vi "应到角度.vi"(1 "目前位置":cluster{"x（cm）":dbl, "y（cm）":dbl, "角度（度）":dbl}, 2 "目标位置":cluster{"x（cm）":dbl, "y（cm）":dbl, "角度（度）":dbl}) -> (0 "应到角度":dbl format="%#_13g")   [LabVIEW 2016]
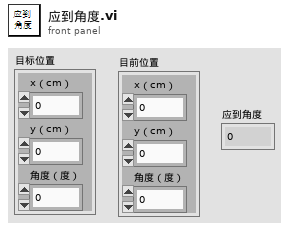
[diagram p1: front panel]
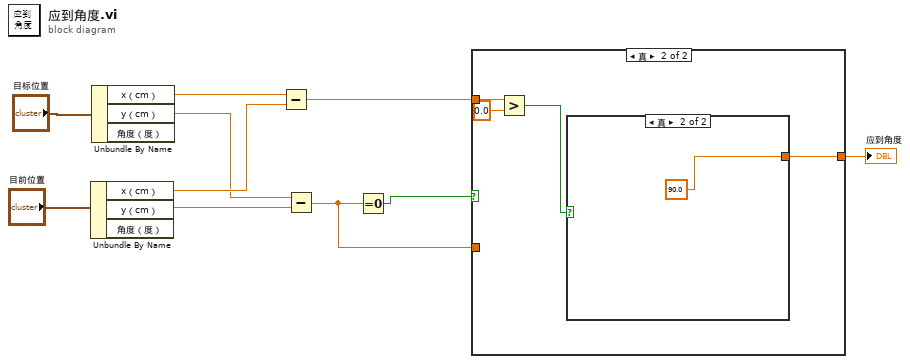
[diagram p0: block diagram]
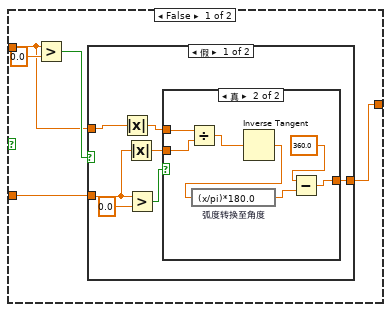
[diagram p2: hidden frame]
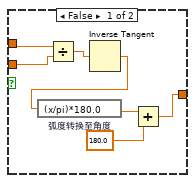
[diagram p3: hidden frame]
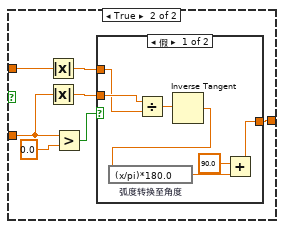
[diagram p4: hidden frame]
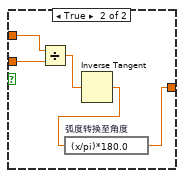
[diagram p5: hidden frame]
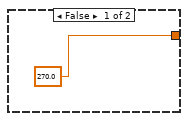
[diagram p6: hidden frame]
diagram:
  n1 = Unbundle By Name("目前位置") -> ("x（cm）"=w7:dbl, "y（cm）"=w5:dbl)  [unwired: 1 out]
  n2 = Unbundle By Name("目标位置") -> ("x（cm）"=w8:dbl, "y（cm）"=w6:dbl)  [unwired: 1 out]
  n3 = Subtract(x=w8, y=w7) -> (x-y=w3:dbl)
  n4 = Subtract(x=w6, y=w5) -> (x-y=w1:dbl)
  n5 = Equal To 0?(x=w1) -> (x = 0?=w4:bool)
  n6 = case shown="真" w4 {
    tunnel: w3 -> [w12 w59]
    tunnel: [w11 w56] -> w2
    tunnel: w1 -> [w13 _]
    frame False {
      n7 = Greater?(x=w12, y=0.0) -> (0:w14:bool)
      n8 = case shown="假" w14 {
        tunnel: w13 -> [w19 w40]
        tunnel: w12 -> [w20 w41]
        tunnel: [w16 w39] -> w11
        frame False {
          n9 = Absolute Value(x=w20) -> (abs(x)=w18:dbl)
          n10 = Absolute Value(x=w19) -> (abs(x)=w17:dbl)
          n11 = Greater?(x=w19, y=0.0) -> (0:w21:bool)
          n12 = case shown="真" w21 {
            tunnel: w18 -> [w29 w36]
            tunnel: w17 -> [w28 w35]
            tunnel: [w23 w30] -> w16
            frame False {
              n13 = Divide(x=w29, y=w28) -> (x/y=w27:dbl)
              n14 = Inverse Tangent(1:w27) -> (0:w26:dbl)
              n15 = expression code="(x/pi)*180.0" "弧度转换至角度"(w26) -> (w25:dbl)
              n16 = Add(x=w25, y=180.0) -> (x+y=w23:dbl)
            }
            frame True {
              n17 = Divide(x=w36, y=w35) -> (x/y=w34:dbl)
              n18 = Inverse Tangent(1:w34) -> (0:w33:dbl)
              n19 = expression code="(x/pi)*180.0" "弧度转换至角度"(w33) -> (w32:dbl)
              n20 = Subtract(x=360.0 ("y"), y=w32) -> (x-y=w30:dbl)
            }
          }
        }
        frame True {
          n21 = Absolute Value(x=w41) -> (abs(x)=w37:dbl)
          n22 = Absolute Value(x=w40) -> (abs(x)=w38:dbl)
          n23 = Greater?(x=w40, y=0.0) -> (0:w42:bool)
          n24 = case shown="假" w42 {
            tunnel: w37 -> [w49 w54]
            tunnel: w38 -> [w50 w55]
            tunnel: [w44 w51] -> w39
            frame False {
              n25 = Divide(x=w50, y=w49) -> (x/y=w48:dbl)
              n26 = Inverse Tangent(1:w48) -> (0:w47:dbl)
              n27 = expression code="(x/pi)*180.0" "弧度转换至角度"(w47) -> (w46:dbl)
              n28 = Add(x=90.0, y=w46) -> (x+y=w44:dbl)
            }
            frame True {
              n29 = Divide(x=w54, y=w55) -> (x/y=w53:dbl)
              n30 = Inverse Tangent(1:w53) -> (0:w52:dbl)
              n31 = expression code="(x/pi)*180.0" "弧度转换至角度"(w52) -> (w51:dbl)
            }
          }
        }
      }
    }
    frame True {
      n32 = Greater?(x=w59, y=0.0) -> (0:w57:bool)
      n33 = case shown="真" w57 {
        tunnel: [270.0 90.0] -> w56
        frame False {
        }
        frame True {
        }
      }
    }
  }
  "应到角度" <- w2
